vi "force_control_ui.vi"(1 "Goal Position IN":sgl[][](array[numeric])) -> (8 "Goal Position OUT":sgl[][](array[numeric]))   [LabVIEW 2014]
uses:
  <vilib>/Analysis/Matrix/Datatypes/RealMatrix.ctl
  <vilib>/Analysis/baseanly.llb/Vector x A.vi
  force_control_globals.vi
  <vilib>/Analysis/Matrix/Numeric/Conversions/Array To Matrix - RA2.vi
  <vilib>/Analysis/Matrix/NI_Matrix.lvlib
  <vilib>/Analysis/NI_AALBase.lvlib
panel:
  out "ASAP to Surface Rotation Matrix":T1
  out "Force Stimulus":dbl[](array[numeric])
  in  "Angle":dbl=0.7
  in  "Rotate FBG Output":bool caption="FBG Enabled"
  in  "FBG Input":dbl[](array[numeric])=[0.0, 0.0, 0.0]
  in  "Override FBG":bool caption="FBG Enabled"
  in  "FBG Scaling":dbl=1.0
  out "FBG Enabled":bool=TRUE
  out "Load Cell Enabled":bool=TRUE
  out "Force Control Active":bool
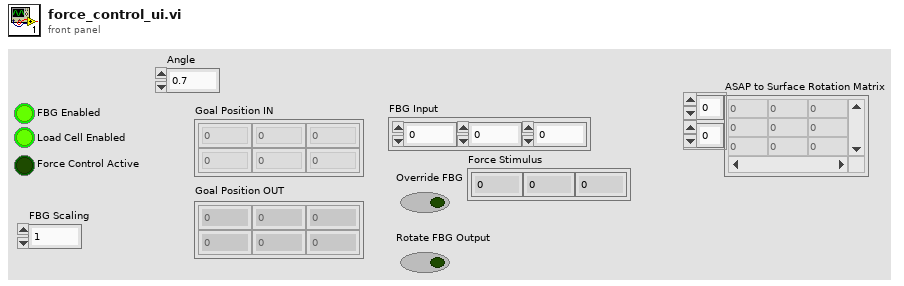
[diagram p1: front panel]
types:
  T1 = typedef "NI_Matrix.lvlib/RealMatrix.ctl" = dbl[][]
  T2 = enum16{"Setpoint", "One Way Threshold", "Two Way Threshold"}
  T3 = enum16{"Translation", "Tip Position", "Rotation"}
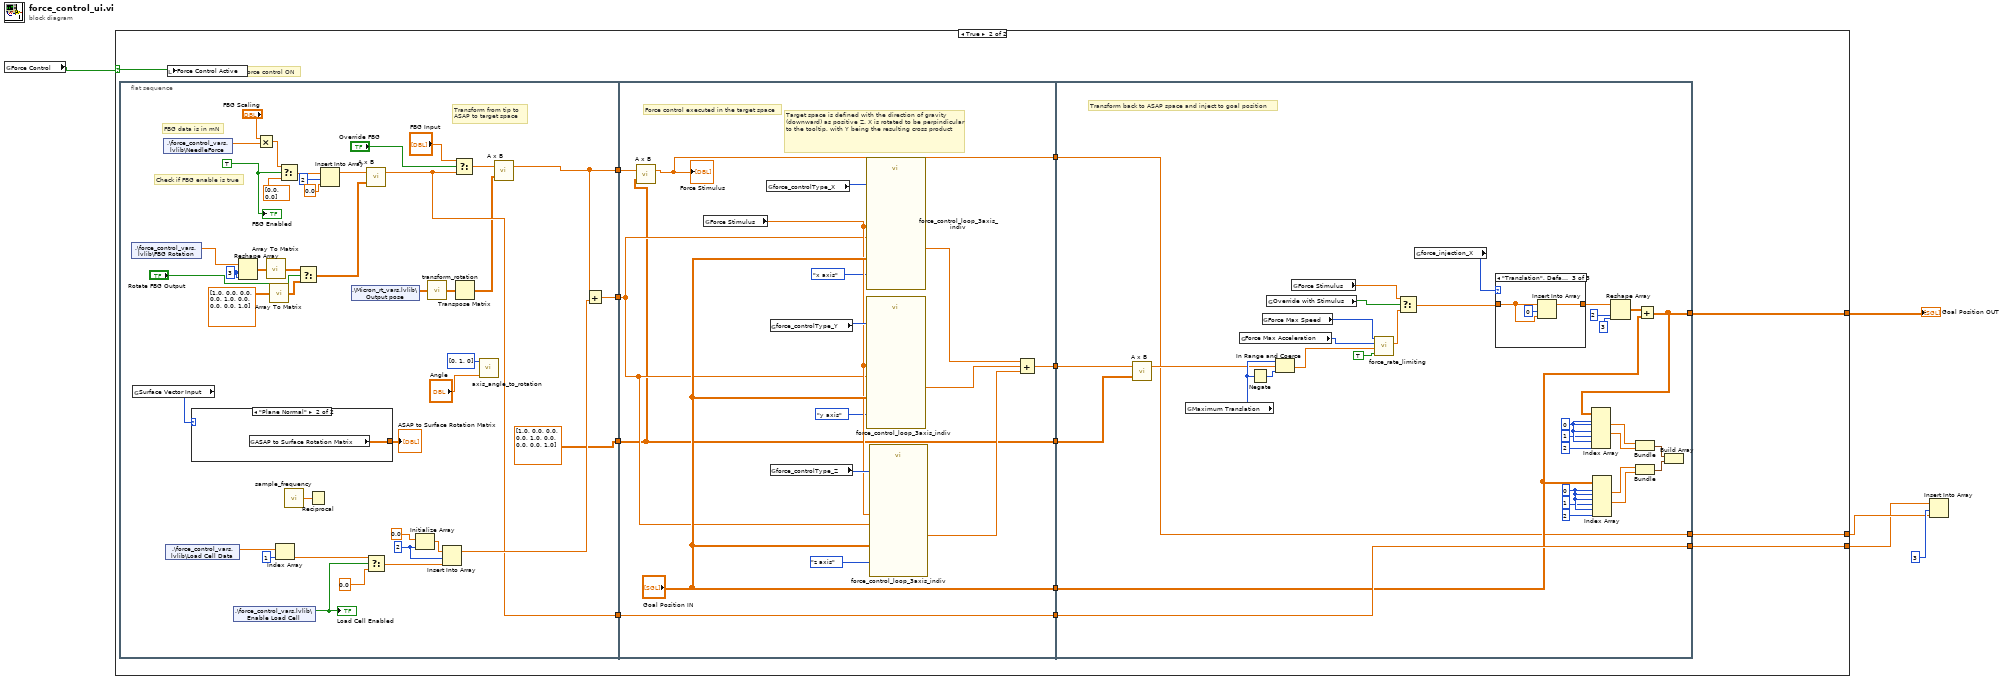
[diagram p0: block diagram]
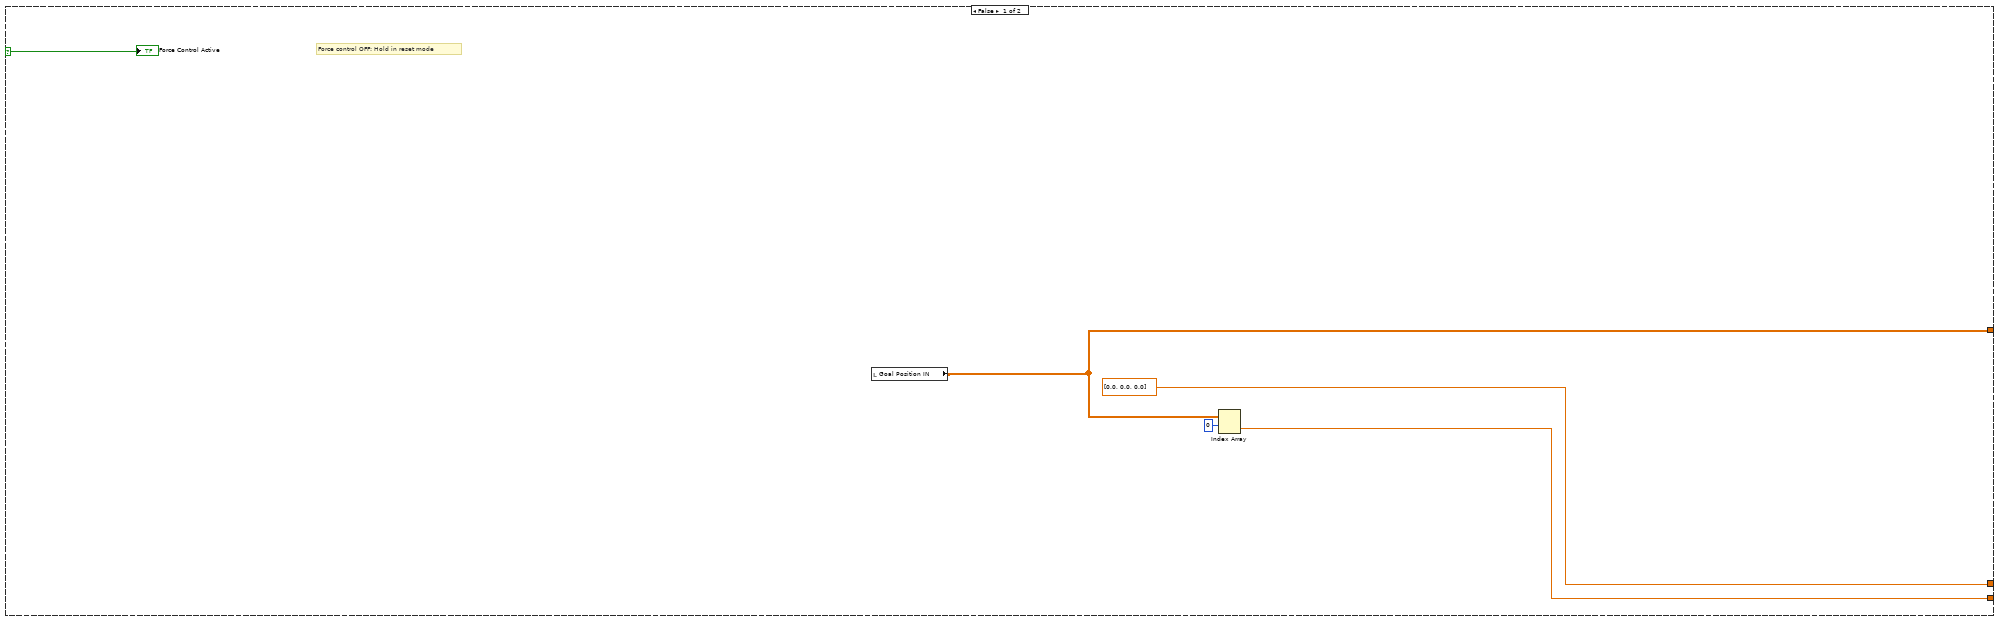
[diagram p2: hidden frame]
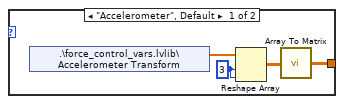
[diagram p3: hidden frame]
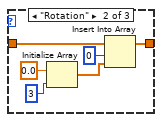
[diagram p5: hidden frame]
diagram:
  n1 = global read "force_control_globals.vi" "Force Control"() -> (w1:bool)
  n2 = case shown="True" w1 {
    selector: w1 -> [w10 w23]
    tunnel: [w6 w22] -> w5
    tunnel: [w8 w16] -> w2
    tunnel: [dbl[] [0.0, 0.0, 0.0] w20] -> w3
    frame False {
      # "Force control OFF: Hold in reset mode"
      n3 = local read "Goal Position IN"() -> (w6:sgl[][])
      n4 = Index Array(array=w6, index (row)=0) -> (element=w8:sgl[])  [unwired: 1 in]
      "Force Control Active" <- w10
    }
    frame True {
      # "Force control ON"
      n5 = flat-sequence {
        tunnel: [w35] -> w21
        tunnel: [w29] -> w14
        tunnel: [w26] -> w13
        tunnel: [dbl[][] [[1.0, 0.0, 0.0], [0.0, 1.0, 0.0], [0.0, 0.0, 1.0]]] -> w11
        tunnel: w21 -> [w77]
        tunnel: [w85] -> w19
        tunnel: [w72] -> w18
        tunnel: [w87] -> w17
        tunnel: ["Goal Position IN"] -> w15
        tunnel: w14 -> [w87]
        tunnel: w13 -> [w73]
        tunnel: [w71] -> w12
        tunnel: w11 -> [w72]
        tunnel: [w105] -> w22
        tunnel: [w100] -> w16
        tunnel: [w88] -> w20
        tunnel: w19 -> [w90]
        tunnel: w18 -> [w92]
        tunnel: w17 -> [w100]
        tunnel: w15 -> [w99]
        tunnel: w12 -> [w88]
        frame #0 {
          w65 = TRUE ("Enable FBG")
          w42 = 3 ("dimension size")
          w61 = 2
          # "Check if FBG enable is true"
          # "FBG data is in mN"
          # "Transform from tip to \nASAP to target space"
          n6 = shared-variable ".\\force_control_vars.lvlib\\FBG Rotation"() -> (w41:dbl[])  [unwired: 1 in, 1 out]
          n7 = global read "force_control_globals.vi" "Surface Vector Input"() -> (w55:enum16{"Accelerometer", "Plane Normal"})
          n8 = shared-variable ".\\force_control_vars.lvlib\\NeedleForce"() -> (w44:dbl[])  [unwired: 1 in, 1 out]
          n9 = shared-variable ".\\force_control_vars.lvlib\\Load Cell Data"() -> (w58:dbl[])  [unwired: 1 in, 1 out]
          n10 = case shown="\"Plane Normal\"" w55 {
            tunnel: [w67 w70] -> w24
            frame "Accelerometer", Default {
              w66 = 3 ("dimension size")
              n11 = shared-variable ".\\force_control_vars.lvlib\\Accelerometer Transform"() -> (w69:dbl[])  [unwired: 1 in, 1 out]
              n12 = Reshape Array(w69, w66, w66) -> (w68:dbl[][])
              n13 = call-poly <vilib>:"Array To Matrix.vi"("Real 2D Array"=w68) -> ("Real Matrix"=w67:T1)
            }
            frame "Plane Normal" {
              n14 = global read "force_control_globals.vi" "ASAP to Surface Rotation Matrix"() -> (w70:T1)
            }
          }
          "ASAP to Surface Rotation Matrix" <- w24
          n15 = shared-variable ".\\force_control_vars.lvlib\\Enable Load Cell"() -> (w59:bool)  [unwired: 1 in, 1 out]
          "Load Cell Enabled" <- w59
          n16 = Reshape Array(w41, w42, w42) -> (w43:dbl[][])
          n17 = Multiply ("Multiply.vi")(x="FBG Scaling", y=w44) -> (x*y=w32:dbl[])
          n18 = call-poly <vilib>:"Array To Matrix.vi"("Real 2D Array"=w43) -> ("Real Matrix"=w40:T1)
          n19 = call-poly <vilib>:"Array To Matrix.vi"("Real 2D Array"=dbl[][] [[1.0, 0.0, 0.0], [0.0, 1.0, 0.0], [0.0, 0.0, 1.0]]) -> ("Real Matrix"=w38:T1)
          n20 = Index Array(array=w58, index=1) -> (element=w49:dbl)
          n21 = Select(t=w32, s=w65, f=sgl[] [0.0, 0.0]) -> (s? t:f=w54:dbl[])
          n22 = call "sample_frequency.vi"() -> ("Sample frequency"=w48:dbl)
          n23 = Select(t=w40, s="Rotate FBG Output", f=w38) -> (s? t:f=w39:T1)
          n24 = Reciprocal(x=w48) -> ()  [unwired: 1 out]
          n25 = Insert Into Array(array=w54, index=2, new element=sgl 0.0 ("new element/subarray")) -> (w30:dbl[])
          n26 = shared-variable ".\\Micron_rt_vars.lvlib\\Output pose"() -> (w64:sgl[][])  [unwired: 1 in, 1 out]
          n27 = call-poly <vilib>:"A x B.vi"("Matrix A"=w39, "Vector V'"=w30) -> ("V' x A"=w29:dbl[])  [unwired: 1 out]
          n28 = Select(t=w49, s=w59, f=0.0 ("lower limit")) -> (s? t:f=w60:dbl)
          n29 = Initialize Array(sgl 0.0, w61) -> (w62:sgl[])
          n30 = call "transform_rotation.vi"("Transform"=w64) -> ("Rotation"=w28:T1)  [unwired: 4 in]
          n31 = Insert Into Array(array=w62, index=w61, new element=w60) -> (w56:sgl[])
          n32 = Select(t="FBG Input", s="Override FBG", f=w29) -> (s? t:f=w31:dbl[])
          n33 = Transpose Matrix(1:w28) -> (0:w27:T1)
          n34 = call "axis_angle_to_rotation.vi"("Angle"="Angle", "Axis"=i32[] [0, 1, 0]) -> ()  [unwired: 9 in, 1 out]
          n35 = call-poly <vilib>:"A x B.vi"("Matrix A"=w27, "Vector V'"=w31) -> ("V' x A"=w26:dbl[])  [unwired: 1 out]
          n36 = Add(x=w26, y=w56) -> (x+y=w35:dbl[])
          "FBG Enabled" <- w65
        }
        frame #1 {
          # "Target space is defined with the direction of gravity (downward) as positive Z. X is rotated to be perpindicular to the tooltip, with Y being the resulting cross product"
          # "Force control executed in the target space"
          n37 = call-poly <vilib>:"A x B.vi"("Matrix A"=w72, "Vector V'"=w73) -> ("V' x A"=w71:dbl[])  [unwired: 1 out]
          "Force Stimulus" <- w71
          n38 = global read "force_control_globals.vi" "Force Stimulus"() -> (w78:dbl[])
          n39 = global read "force_control_globals.vi" "force_controlType_X"() -> (w86:T2)
          n40 = global read "force_control_globals.vi" "force_controlType_Y"() -> (w79:T2)
          n41 = global read "force_control_globals.vi" "force_controlType_Z"() -> (w80:T2)
          n42 = call "force_control_loop_3axis_indiv.vi"("Force In"=w77, "Goal Position IN"="Goal Position IN", "Force Stimulus"=w78, "Control Axis"=enum16{"x axis", "y axis", "z axis"}."x axis", "Force Control Type"=w86) -> ("Force Position Out"=w84:dbl[])  [unwired: 9 in, 1 out]
          n43 = call "force_control_loop_3axis_indiv.vi"("Force In"=w77, "Goal Position IN"="Goal Position IN", "Force Stimulus"=w78, "Control Axis"=enum16{"x axis", "y axis", "z axis"}."y axis", "Force Control Type"=w79) -> ("Force Position Out"=w83:dbl[])  [unwired: 9 in, 1 out]
          n44 = call "force_control_loop_3axis_indiv.vi"("Force In"=w77, "Goal Position IN"="Goal Position IN", "Force Stimulus"=w78, "Control Axis"=enum16{"x axis", "y axis", "z axis"}."z axis", "Force Control Type"=w80) -> ("Force Position Out"=w82:dbl[])  [unwired: 9 in, 1 out]
          n45 = Compound Arithmetic op=ADD(w84, w83, w82) -> (w85:dbl[])
        }
        frame #2 {
          w112 = 0 ("index")
          w116 = 0 ("index")
          # "Transform back to ASAP space and inject to goal position"
          n46 = call-poly <vilib>:"A x B.vi"("Matrix A"=w92, "Vector V'"=w90) -> ("V' x A"=w89:dbl[])  [unwired: 1 out]
          n47 = global read "force_control_globals.vi" "Maximum Translation"() -> (w95:i32)
          n48 = global read "force_control_globals.vi" "Force Max Acceleration"() -> (w97:i32)
          n49 = Negate(x=w95) -> (-x=w104:i32)
          n50 = global read "force_control_globals.vi" "Force Max Speed"() -> (w98:i32)
          n51 = global read "force_control_globals.vi" "Override with Stimulus"() -> (w96:bool)
          n52 = In Range and Coerce(upper limit=w95, x=w89, lower limit=w104) -> (coerced(x)=w103:dbl[])  [unwired: 1 out]
          n53 = global read "force_control_globals.vi" "Force Stimulus"() -> (w91:dbl[])
          n54 = call "force_rate_limiting.vi"("Rate Limiting"=TRUE, "Link goal"=w103, "force max accel"=w97, "force max vel"=w98) -> ("Substituted goal"=w101:sgl[])  [unwired: 7 in]
          n55 = Select(t=w91, s=w96, f=w101) -> (s? t:f=w93:dbl[])
          n56 = global read "force_control_globals.vi" "force_injection_X"() -> (w94:T3)
          n57 = case shown="\"Translation\", Default" w94 {
            tunnel: [w122 w127 w130] -> w119
            tunnel: w93 -> [w122 w126 w129]
            frame "Tip Position" {
            }
            frame "Rotation" {
              n58 = Initialize Array(0.0 ("element"), 3 ("dimension size")) -> (w125:dbl[])
              n59 = Insert Into Array(array=w126, index=0, new element=w125) -> (w127:dbl[])
            }
            frame "Translation", Default {
              n60 = Insert Into Array(array=w129, index=0, new element=w129) -> (w130:dbl[])
            }
          }
          n61 = Index Array(array=w99, index (row) #1=w112, index (col) #1=w112, index (row) #2=w112, index (col) #2=1 ("length"), index (row) #3=w112, index (col) #3=2 ("length")) -> (element #1=w108:sgl, element #2=w107:sgl)  [unwired: 1 out]
          n62 = Reshape Array(w119, 2, 3) -> (w106:dbl[][])
          n63 = Bundle("Numeric"=w108, "Numeric"=w107) -> (w118:cluster{"Numeric":sgl, "Numeric":sgl})  [unwired: 1 in]
          n64 = Add ("Add.vi")(x=w106, y=w99) -> (x+y=w105:dbl[][])
          n65 = Index Array(array=w105, index (row) #1=w116, index (col) #1=w116, index (row) #2=w116, index (col) #2=1 ("length"), index (row) #3=w116, index (col) #3=2 ("length")) -> (element #1=w110:dbl, element #2=w109:dbl)  [unwired: 1 out]
          n66 = Bundle(w110, w109) -> (w117:cluster{dbl, dbl})  [unwired: 1 in]
          n67 = Build Array(w117, w118) -> ()  [unwired: 1 out]
        }
      }
      n68 = local write "Force Control Active"(w23) -> ()
    }
  }
  "Goal Position OUT" <- w5
  n69 = Insert Into Array(array=w2, index=3, new element=w3) -> ()  [unwired: 1 out]
